vi "Conventional_DSB(SubVI).vi"(4 "mod index":dbl(slide)=1.0 scale=0.0..1.0, 5 "modulation frequency":dbl(knob)=10.0 scale=0.0..1000.0, 6 "sampling info":cluster{"Fs":dbl, "#s":dbl}, 7 "carrier frequency":dbl(knob)=10.0 scale=0.0..500000.0) -> (0 "baseband signal (time-domain)":waveform(dbl)(graph), 1 "baseband signal (frequency-domain)":cluster{"f0":dbl, "df":dbl, "magnitude":dbl[]}(graph), 2 "Baseband/AM":dbl, 3 "modulated signal (time-domain)":waveform(dbl)(graph))   [LabVIEW 2010]
uses:
  <vilib>/measure/maspectr.llb/FFT Spectrum (Mag-Phase) for 1 Chan.vi
  <vilib>/measure/NI_MABase.lvlib
  <vilib>/measure/NI_MAPro.lvlib
  <vilib>/ptbypt/NI_PtbyPt.lvlib
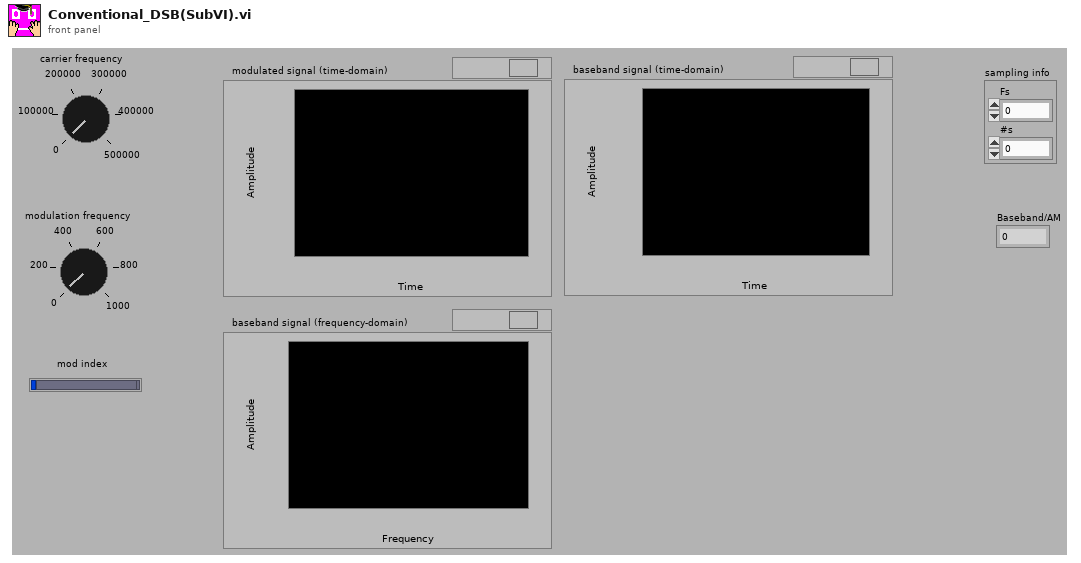
[diagram p1: front panel]
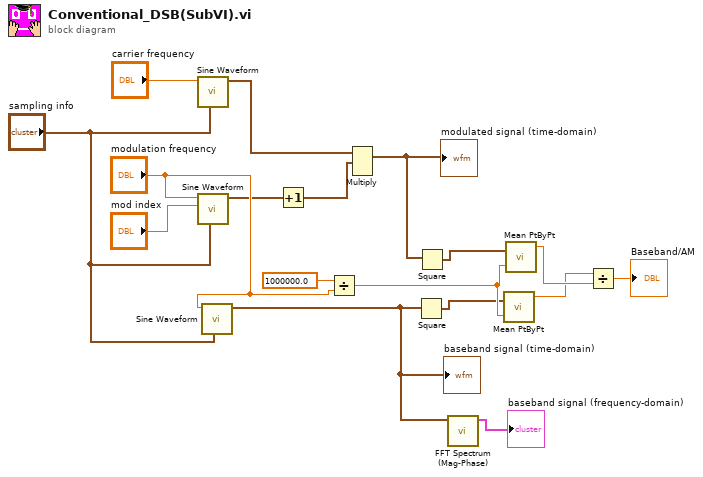
[diagram p0: block diagram]
diagram:
  n1 = call <vilib>:"Sine Waveform.vi"("sampling info"="sampling info", "frequency"="carrier frequency") -> ("signal out"=w3:waveform(dbl))  [unwired: 8 in, 1 out]
  n2 = call <vilib>:"Sine Waveform.vi"("sampling info"="sampling info", "amplitude"="mod index", "frequency"="modulation frequency") -> ("signal out"=w12:waveform(dbl))  [unwired: 7 in, 1 out]
  n3 = call <vilib>:"Sine Waveform.vi"("sampling info"="sampling info", "frequency"="modulation frequency") -> ("signal out"=w15:waveform(dbl))  [unwired: 8 in, 1 out]
  "baseband signal (time-domain)" <- w15
  n4 = Increment(x=w12) -> (x+1=w4:waveform(dbl))
  n5 = Divide(x=1000000.0, y="modulation frequency") -> (x/y=w10:dbl)
  n6 = Multiply(1:w4, 2:w3) -> (0:w6:waveform(dbl))  [unwired: 1 in, 1 out]
  "modulated signal (time-domain)" <- w6
  n7 = Square(x=w15) -> (x^2=w7:waveform(dbl))
  n8 = Square(x=w6) -> (x^2=w8:waveform(dbl))
  n9 = call-poly <vilib>:"FFT Spectrum (Mag-Phase).vi"("time signal"=w15) -> ("magnitude"=→"baseband signal (frequency-domain)":cluster{"f0":dbl, "df":dbl, "magnitude":dbl[]})  [unwired: 6 in, 4 out]
  n10 = call <vilib>:"Mean PtByPt.vi"("x"=w7, "sample length"=w10) -> ("mean"=w13:dbl)  [unwired: 2 in, 1 out]
  n11 = call <vilib>:"Mean PtByPt.vi"("x"=w8, "sample length"=w10) -> ("mean"=w14:dbl)  [unwired: 2 in, 1 out]
  n12 = Divide(x=w13, y=w14) -> (x/y=→"Baseband/AM":dbl)
